vi "Hilfe.vi"   [LabVIEW 2020, in "EPA 1065.lvlib" / "Interference verificaton 1065-366.lvlib"]
uses:
  Interference verificaton 1065-366.lvlib
  Allgemein/allgemeine Sub-VIs.lvlib
panel:
  # "Toleranzbereich für Start der Messaufzeichung. Betrifft Komponenten- und H²O Konzentration. Empfohlen 5%. Bei dem Wert 0 wird eine 10 Sekunden Zeitverzögerung angewandt."
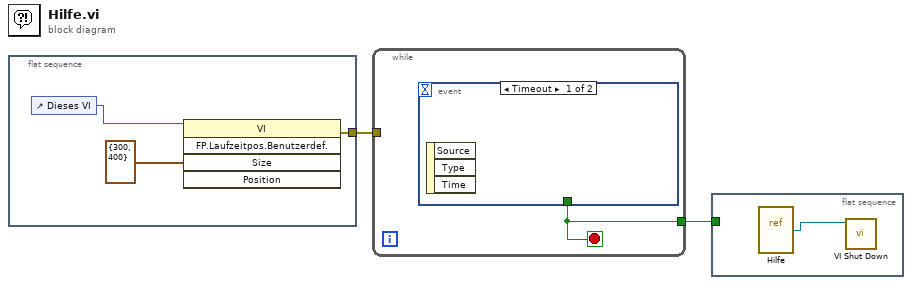
[diagram p0: block diagram]
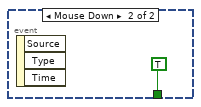
[diagram p2: hidden frame]
diagram:
  n1 = flat-sequence {
    tunnel: [w3] -> w1
    frame #0 {
      n2 = control-ref of="Dieses VI"() -> (w4:refnum<vi>)
      n3 = invoke class="VI" method="FP.Laufzeitpos.Benutzerdef."(reference=w4, "Size"=cluster{"Top":i16, "Left":i16} {"Top"=300, "Left"=400} ("Position")) -> (error out=w3:errorcluster)  [unwired: 3 in, 4 out]
    }
  }
  n4 = while {
    tunnel: [w6] -> w2
    tunnel: w1 -> [_]
    stop <- w6 stop-if-true
    n5 = event shown="[0] Timeout" {
      selector: _ -> [_ _]
      dyn-events: _ -> [_ _]
      timeout: _ -> [_ _]
      tunnel: [_ TRUE] -> w6
      event Timeout {
        n6 = event-data() -> ()  [unwired: 1 in, 3 out]
      }
      event Mouse Down {
        n7 = event-data() -> ()  [unwired: 1 in, 3 out]
      }
    }
  }
  n8 = flat-sequence {
    tunnel: w2 -> [_]
    frame #0 {
      n9 = vi-ref "Hilfe.vi"() -> (w8:refnum<vi>)
      n10 = call "VI Shut Down.vi"("VI Referenz"=w8) -> ()  [unwired: 11 in]
    }
  }
